vi "write_data.vi"(8 "error in (no error)":errorcluster, 10 "data":T1, 11 "TweedieRegressor in":refnum<class "TweedieRegressor.lvclass">) -> (0 "error out":errorcluster, 3 "TweedieRegressor out":refnum<class "TweedieRegressor.lvclass">)   [LabVIEW 2020, in "TweedieRegressor.lvclass"]
uses:
  TweedieRegressor.lvclass
  Controls/tweedie_regressor_data.ctl
  TweedieRegressor.lvclass/TweedieRegressor.ctl
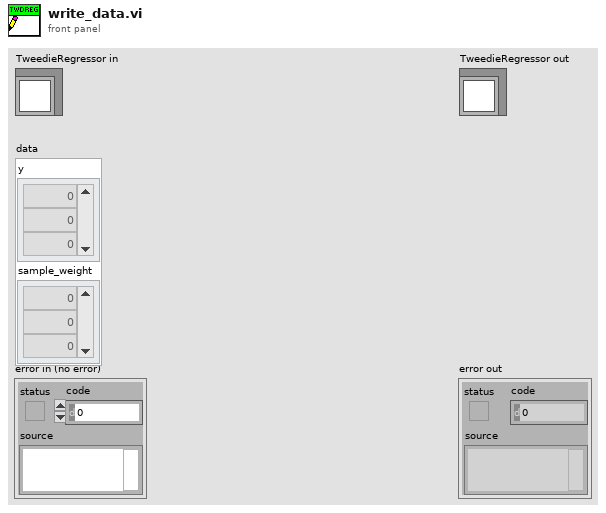
[diagram p1: front panel]
types:
  T1 = typedef "tweedie_regressor_data.ctl" = cluster{"y":dbl[], "sample_weight":dbl[]}
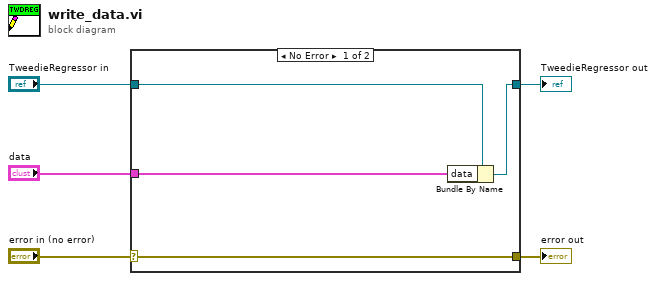
[diagram p0: block diagram]
diagram:
  n1 = case shown="No Error" "error in (no error)" {
    selector: "error in (no error)" -> [w9 w10]
    tunnel: [w9 w10] -> w4
    tunnel: [w7 w11] -> w2
    tunnel: "TweedieRegressor in" -> [w8 w11]
    tunnel: "data" -> [w6 _]
    frame No Error {
      n2 = Bundle By Name(cluster=w8, "data"=w6) -> (w7:refnum<class "TweedieRegressor.lvclass">)
    }
    frame Error {
    }
  }
  "error out" <- w4
  "TweedieRegressor out" <- w2
